vi "Configure Measurement.vi"(6 "Manual Range (1.0)":dbl=1.0, 8 "error in (no error)":errorcluster, 9 "Enable Auto Range (T:Enable)":bool=TRUE, 10 "Function (0: Volts)":u16(ring) items=["Volts", "Current", "Resistance"], 11 "VISA resource name":refnum<visa-resource-name>) -> (0 "error out":errorcluster, 3 "VISA resource name out":refnum<visa-resource-name>)   [LabVIEW 2018, in "Keithley 24XX.lvlib"]
doc: "Configures the measurement type, resolution, and range on the instrument.\n\n<B>Note:</B> This VI should be called for each measurement that is of interest. This VI can be called multiple times in a row."
uses:
  Keithley 24XX.lvlib
panel:
  out "String":string
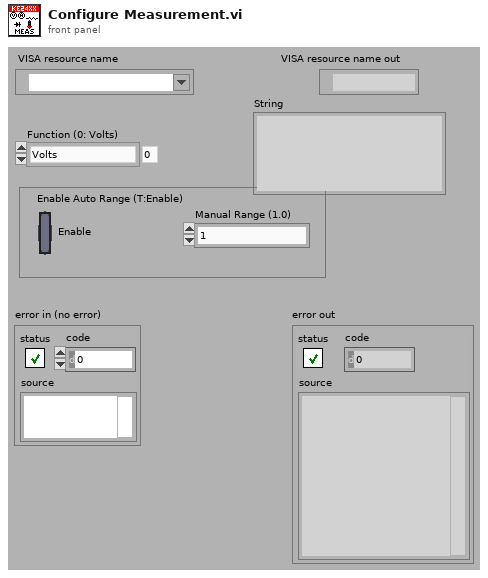
[diagram p1: front panel]
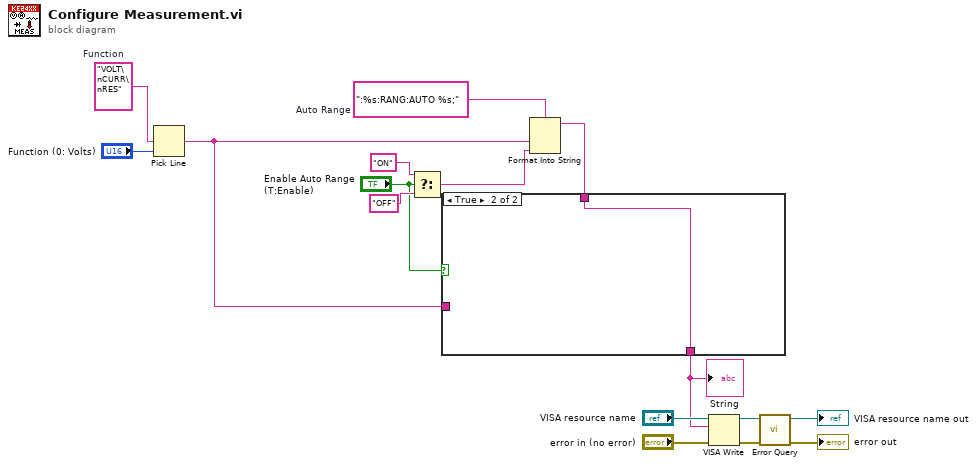
[diagram p0: block diagram]
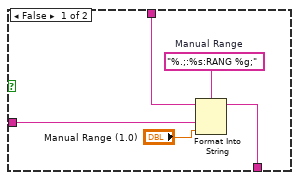
[diagram p2: hidden frame]
diagram:
  w8 = ":%s:RANG:AUTO %s;"  # Auto Range
  w12 = "VOLT\nCURR\nRES"  # Function
  n1 = Pick Line(multi-line string=w12, line index="Function (0: Volts)") -> (output string=w7:string)  [unwired: 1 in]
  n2 = Select(t="ON", s="Enable Auto Range (T:Enable)", f="OFF") -> (s? t:f=w4:string)
  n3 = Format Into String(format string=w8, w7, w4) -> (resulting string=w3:string)  [unwired: 2 in, 1 out]
  n4 = case shown="True" "Enable Auto Range (T:Enable)" {
    tunnel: w7 -> [w19 _]
    tunnel: w3 -> [w18 w22]
    tunnel: [w17 w22] -> w2
    frame False {
      w21 = "%.;:%s:RANG %g;"  # Manual Range
      n5 = Format Into String(format string=w21, initial string=w18, w19, "Manual Range (1.0)") -> (resulting string=w17:string)  [unwired: 1 in, 1 out]
    }
    frame True {
    }
  }
  "String" <- w2
  n6 = VISA Write(VISA resource name="VISA resource name", write buffer=w2, error in (no error)="error in (no error)") -> (VISA resource name out=w10:refnum<visa-resource-name>, error out=w9:errorcluster)  [unwired: 1 out]
  n7 = call "Error Query.vi"("error in (no error)"=w9, "VISA resource name"=w10) -> ("error out"=→"error out":errorcluster, "VISA resource name out"=→"VISA resource name out":refnum<visa-resource-name>)  [unwired: 6 in, 2 out]
